vi "Sort_IntString.vi"(7 "Array_Int_IN":i32[](array[numeric]), 10 "Array - String_IN":string[](array[string])) -> (3 "Array_String_OUT":string[][](array[string]))   [LabVIEW 2020]
doc: "Sortuje iloœæ wybranych opcji w formacie INT 32, nastêpnie zamienia te liczby na format String."
uses:
  d97d2a8e-1911-4199-bd68-117c03c96036.vi
  <vilib>/Comparison/Less/Less Functor/Less Functor.lvclass
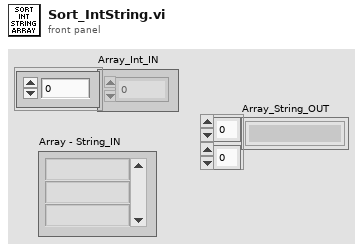
[diagram p1: front panel]
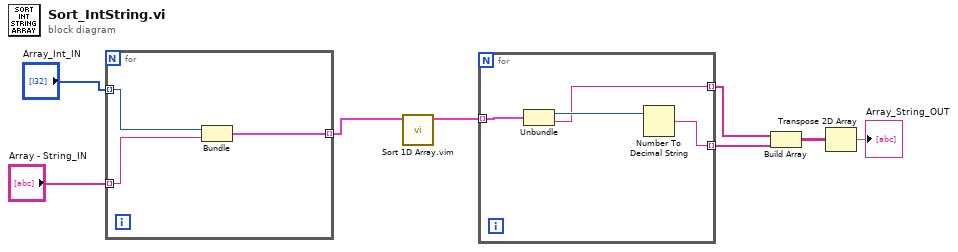
[diagram p0: block diagram]
diagram:
  n1 = for {
    tunnel: "Array_Int_IN" -> [w11] mode=indexing
    tunnel: "Array - String_IN" -> [w10] mode=indexing
    tunnel: [w9] -> w6 mode=indexing
    n2 = Bundle("Numeric"=w11, "String"=w10) -> (w9:cluster{"Numeric":i32, "String":string})  [unwired: 1 in]
  }
  n3 = call "Sort 1D Array.vim"("unsorted array"=w6) -> ("sorted array"=w5:cluster{"Numeric":i32, "String":string}[])  [unwired: 10 in]
  n4 = for {
    tunnel: w5 -> [w15] mode=indexing
    tunnel: [w13] -> w4 mode=indexing
    tunnel: [w12] -> w3 mode=indexing
    n5 = Unbundle(w15) -> ("Numeric"=w14:i32, "String"=w13:string)
    n6 = Number To Decimal String(number=w14) -> (decimal integer string=w12:string)  [unwired: 1 in]
  }
  n7 = Build Array(w4, w3) -> (w2:string[][])
  n8 = Transpose 2D Array(2D array=w2) -> (transposed array=→"Array_String_OUT":string[][])
